vi "Yattzee.vi"() -> ()   [LabVIEW 2022 SP3]
uses:
  <vilib>/numeric/Random Number (Range) U64.vi
  <vilib>/numeric/sub_Random U32.vi
panel:
  out "concatenated string":string
  out "26-35":bool
  out "16-25":bool
  out "6-15":bool
  out "Numeric 6":dbl
  out "Numeric 5":dbl
  out "Numeric 4":dbl
  out "Numeric 3":dbl
  out "Numeric 2":dbl
  out "Numeric":dbl
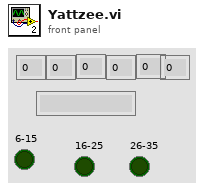
[diagram p1: front panel]
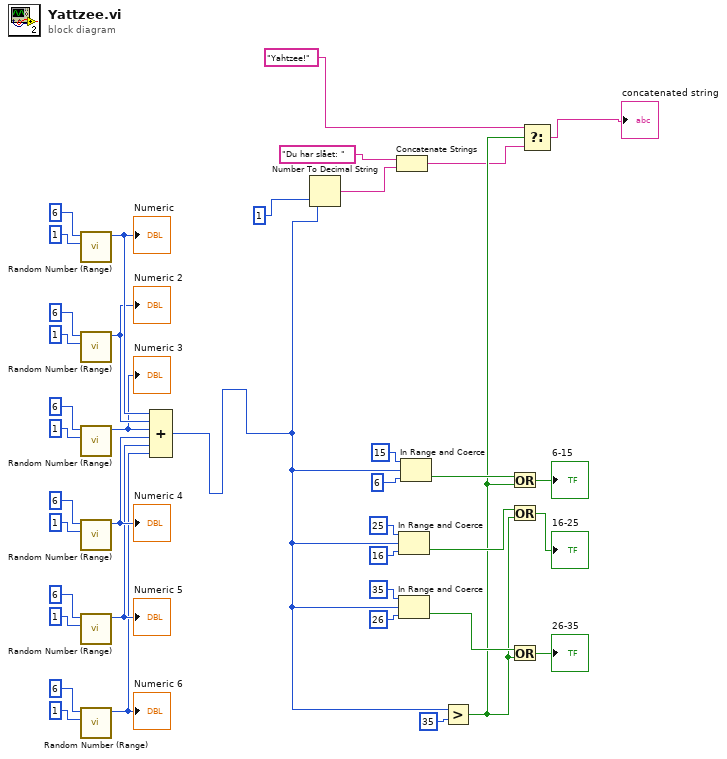
[diagram p0: block diagram]
diagram:
  n1 = call-poly <vilib>:"Random Number (Range).vi"("lower bound (0)"=u64 1, "upper bound (100)"=u64 6) -> ("number"=w27:u64)  [unwired: 9 in]
  "Numeric" <- w27
  n2 = call-poly <vilib>:"Random Number (Range).vi"("lower bound (0)"=u64 1, "upper bound (100)"=u64 6) -> ("number"=w26:u64)  [unwired: 9 in]
  "Numeric 2" <- w26
  n3 = call-poly <vilib>:"Random Number (Range).vi"("lower bound (0)"=u64 1, "upper bound (100)"=u64 6) -> ("number"=w25:u64)  [unwired: 9 in]
  "Numeric 3" <- w25
  n4 = call-poly <vilib>:"Random Number (Range).vi"("lower bound (0)"=u64 1, "upper bound (100)"=u64 6) -> ("number"=w24:u64)  [unwired: 9 in]
  "Numeric 4" <- w24
  n5 = call-poly <vilib>:"Random Number (Range).vi"("lower bound (0)"=u64 1, "upper bound (100)"=u64 6) -> ("number"=w23:u64)  [unwired: 9 in]
  "Numeric 5" <- w23
  n6 = call-poly <vilib>:"Random Number (Range).vi"("lower bound (0)"=u64 1, "upper bound (100)"=u64 6) -> ("number"=w22:u64)  [unwired: 9 in]
  "Numeric 6" <- w22
  n7 = Compound Arithmetic op=ADD(w27, w26, w25, w24, w23, w22) -> (w2:u64)
  n8 = Number To Decimal String(number=w2, width (-)=i16 1) -> (decimal integer string=w8:string)
  n9 = Concatenate Strings("Du har slået: " ("string"), w8) -> (w4:string)
  n10 = In Range and Coerce(upper limit=u64 25 ("lower limit"), x=w2, lower limit=u64 16 ("upper limit")) -> (In Range?=w20:bool)  [unwired: 1 out]
  n11 = In Range and Coerce(upper limit=u64 35 ("lower limit"), x=w2, lower limit=u64 26 ("upper limit")) -> (In Range?=w19:bool)  [unwired: 1 out]
  n12 = In Range and Coerce(upper limit=u64 15 ("lower limit"), x=w2, lower limit=u64 6 ("upper limit")) -> (In Range?=w10:bool)  [unwired: 1 out]
  n13 = Greater?(x=w2, y=u64 35 ("lower limit")) -> (0:w6:bool)
  n14 = Or(x=w10, y=w6) -> (x .or. y?=→"6-15":bool)
  n15 = Or(x=w20, y=w6) -> (x .or. y?=→"16-25":bool)
  n16 = Or(x=w19, y=w6) -> (x .or. y?=→"26-35":bool)
  n17 = Select(t="Yahtzee!" ("f"), s=w6, f=w4) -> (s? t:f=→"concatenated string":string)
